vi "getStatus.vi"(8 "error in (no error)":errorcluster, 9 "Monochromator in":refnum<class "Monochromator.lvclass">, 11 "SettingUpState in":refnum<class "SettingUpState.lvclass">) -> (0 "error out":errorcluster, 1 "Monochromator out":refnum<class "Monochromator.lvclass">, 2 "DeviceStatus":T1, 3 "SettingUpState out":refnum<class "SettingUpState.lvclass">)   [LabVIEW 2016, in "SettingUpState.lvclass"]
uses:
  SettingUpState.lvclass
  Monochromator/Monochromator.lvclass
  Typedefs/DeviceStatus.ctl
  Monochromator/Monochromator.lvclass/Monochromator.ctl
  MonoCommunicator/MonoCommunicator.lvclass
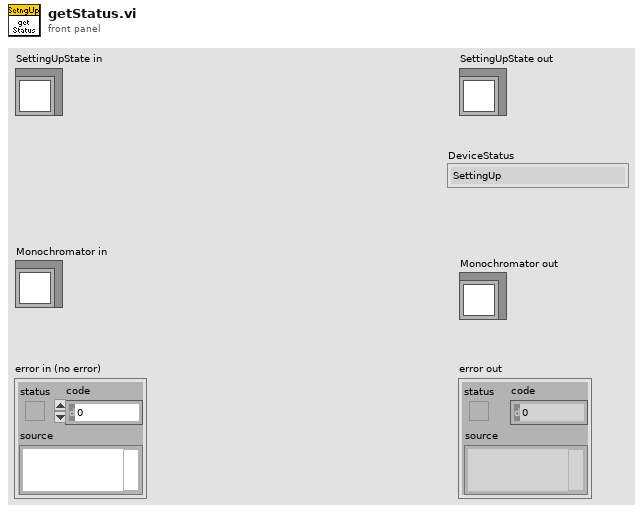
[diagram p1: front panel]
types:
  T1 = typedef "DeviceStatus.ctl" = enum16{"SettingUp", "Ready", "Offline", "Fault"}
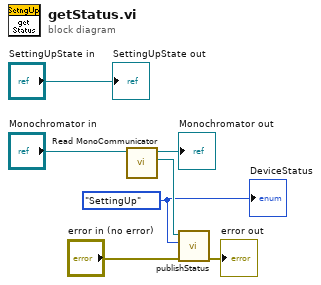
[diagram p0: block diagram]
diagram:
  w1 = DeviceStatus."SettingUp" ("DeviceStatus")
  n1 = call "Read MonoCommunicator.vi"("Monochromator in"="Monochromator in") -> ("MonoCommunicator.lvclass"=w2:refnum<class "MonoCommunicator.lvclass">, "Monochromator out"=→"Monochromator out":refnum<class "Monochromator.lvclass">)  [unwired: 8 in, 1 out]
  n2 = call "publishStatus.vi"("error in (no error)"="error in (no error)", "DeviceStatus"=w1, "MonoCommunicator in"=w2) -> ("error out"=→"error out":errorcluster)  [unwired: 7 in, 1 out]
  "SettingUpState out" <- "SettingUpState in"
  "DeviceStatus" <- w1
